vi "Sequence.BuildWaveform.vi"(10 "Steps":string[][](array[string]), 11 "Duration":string[](array[string])) -> (3 "Array":waveform(dbl)[](array[waveform]))   [LabVIEW 2013, in "Simple Sequence Tools - Shared.lvlib"]
uses:
  Simple Sequence Tools - Shared.lvlib
  <vilib>/Analysis/1siggen.llb/Ramp Pattern by Samples.vi
  <vilib>/Analysis/1siggen.llb/Ramp Pattern by Delta.vi
  <vilib>/Analysis/NI_AALBase.lvlib
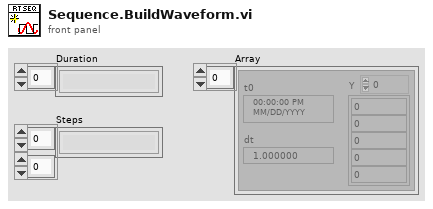
[diagram p1: front panel]
types:
  T1 = typedef "Simple Sequence Tools - Shared.lvlib/StepTypes.ctl" = enum8{"Step", "iStep", "Ramp", "Unchanged", "Unknown"}
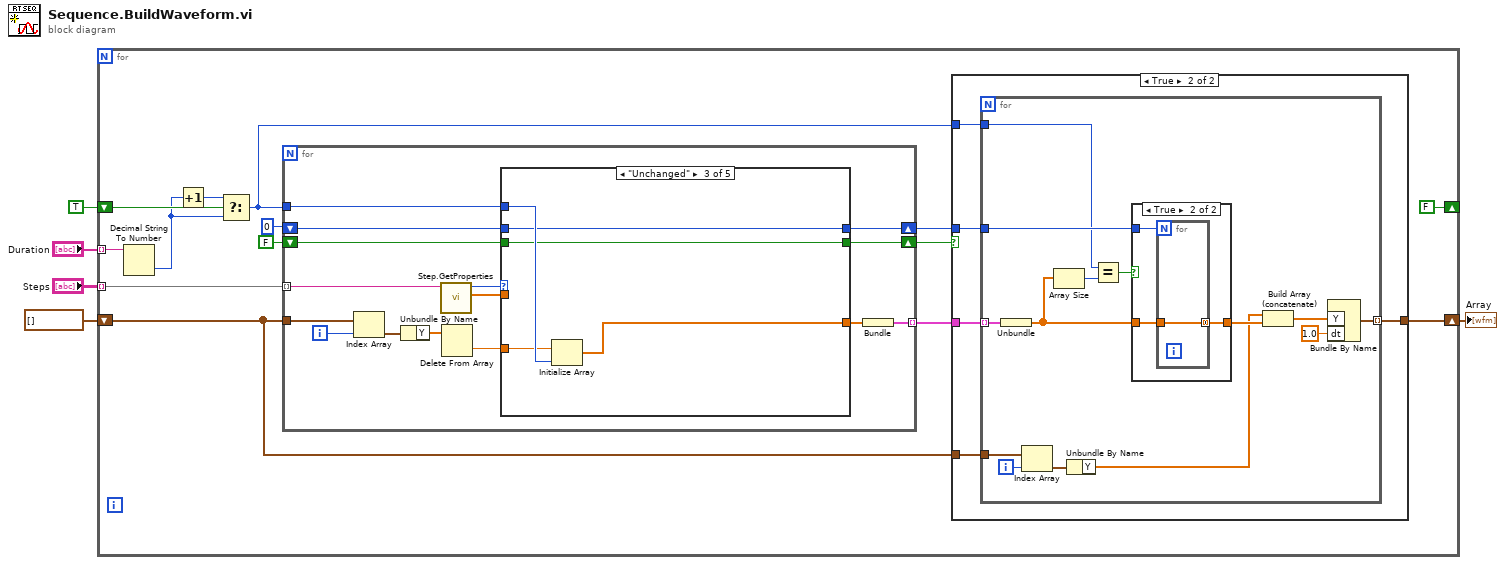
[diagram p0: block diagram]
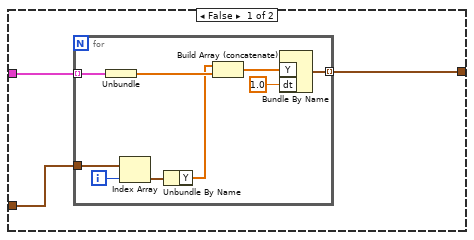
[diagram p2: hidden frame]
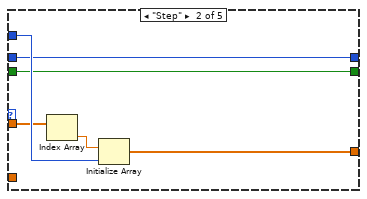
[diagram p5: hidden frame]
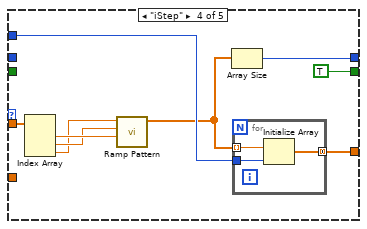
[diagram p6: hidden frame]
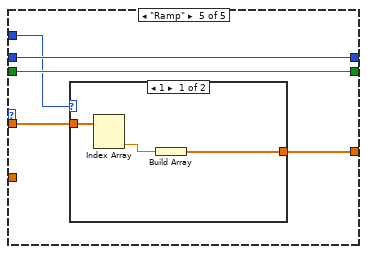
[diagram p7: hidden frame]
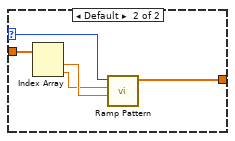
[diagram p8: hidden frame]
diagram:
  n1 = for {
    tunnel: "Steps" -> [w19] mode=indexing
    tunnel: "Duration" -> [w18] mode=indexing
    shift-right: [FALSE] -> _
    shift-left: TRUE -> [w11]
    shift-right: [w7] -> w1
    shift-left: waveform(dbl)[] [] -> [w6]
    n2 = Decimal String To Number(string=w18) -> (number=w10:i32)  [unwired: 2 in, 1 out]
    n3 = Increment(x=w10) -> (x+1=w9:i32)
    n4 = Select(t=w9, s=w11, f=w10) -> (s? t:f=w8:i32)
    n5 = for {
      tunnel: w19 -> [w70] mode=indexing
      tunnel: w8 -> [w68]
      shift-right: [w65] -> w15
      shift-left: FALSE -> [w66]
      shift-right: [w63] -> w14
      shift-left: 0 -> [w62]
      tunnel: [w61] -> w13 mode=indexing
      tunnel: w6 -> [w60]
      i -> [w58]
      n6 = Index Array(array=w60, index=w58) -> (element=w57:waveform(dbl))
      n7 = Unbundle By Name(w57) -> ("Y"=w56:dbl[])
      n8 = call "Step.GetProperties.vi"("String in"=w70) -> ("Parameters"=w67:dbl[], "Step"=w69:T1)  [unwired: 8 in, 1 out]
      n9 = Delete From Array(array=w56) -> (deleted portion=w59:dbl)  [unwired: 2 in, 1 out]
      n10 = case shown="\"Unchanged\"" w69 {
        tunnel: w68 -> [_ w78 w83 w91 w96]
        tunnel: w67 -> [_ w77 _ w92 w100]
        tunnel: [_ w75 w82 w86 w99] -> w64
        tunnel: w66 -> [w72 w74 w81 _ w98]
        tunnel: [w72 w74 w81 TRUE w98] -> w65
        tunnel: [w71 w73 w80 w84 w97] -> w63
        tunnel: w62 -> [w71 w73 w80 _ w97]
        tunnel: w59 -> [_ _ w79 _ _]
        frame Default {
        }
        frame "Step" {
          n11 = Index Array(array=w77) -> (element=w76:dbl)  [unwired: 1 in]
          n12 = Initialize Array(w76, w78) -> (w75:dbl[])
        }
        frame "Unchanged" {
          n13 = Initialize Array(w79, w83) -> (w82:dbl[])
        }
        frame "iStep" {
          n14 = Index Array(array=w92) -> (element #1=w90:dbl, element #2=w89:dbl, element #3=w88:dbl)  [unwired: 3 in]
          n15 = call-poly <vilib>:"Ramp Pattern.vi"("start"=w90, "end"=w89, "delta"=w88) -> ("Ramp Pattern"=w85:dbl[])  [unwired: 6 in, 2 out]
          n16 = Array Size(array=w85) -> (size(s)=w84:i32)
          n17 = for {
            tunnel: w91 -> [w95]
            tunnel: w85 -> [w94] mode=indexing
            tunnel: [w93] -> w86 mode=concatenating
            n18 = Initialize Array(w94, w95) -> (w93:dbl[])
          }
        }
        frame "Ramp" {
          n19 = case shown="1" w96 {
            selector: w96 -> [_ w104]
            tunnel: w100 -> [w103 w108]
            tunnel: [w101 w105] -> w99
            frame 1 {
              n20 = Index Array(array=w103) -> (element #2=w102:dbl)  [unwired: 2 in, 1 out]
              n21 = Build Array(w102) -> (w101:dbl[])
            }
            frame Default {
              n22 = Index Array(array=w108) -> (element #1=w107:dbl, element #2=w106:dbl)  [unwired: 2 in]
              n23 = call-poly <vilib>:"Ramp Pattern.vi"("start"=w107, "end"=w106, "samples"=w104) -> ("Ramp Pattern"=w105:dbl[])  [unwired: 7 in, 1 out]
            }
          }
        }
      }
      n24 = Bundle("Ramp Pattern"=w64) -> (w61:cluster{"Ramp Pattern":dbl[]})  [unwired: 1 in]
    }
    n25 = case shown="True" w15 {
      tunnel: w14 -> [_ w35]
      tunnel: w13 -> [w22 w36]
      tunnel: w8 -> [_ w34]
      tunnel: [w21 w33] -> w7
      tunnel: w6 -> [w20 w32]
      frame False {
        n26 = for {
          tunnel: w22 -> [w31] mode=indexing
          tunnel: [w29] -> w21 mode=indexing
          tunnel: w20 -> [w24]
          i -> [w25]
          n27 = Unbundle(w31) -> ("Ramp Pattern"=w28:dbl[])
          n28 = Index Array(array=w24, index=w25) -> (element=w23:waveform(dbl))
          n29 = Unbundle By Name(w23) -> ("Y"=w26:dbl[])
          n30 = Build Array (concatenate)(w26, w28) -> (w27:dbl[])
          n31 = Bundle By Name("Y"=w27, "dt"=1.0) -> (w29:waveform(dbl))  [unwired: 1 in]
        }
      }
      frame True {
        n32 = for {
          tunnel: w36 -> [w49] mode=indexing
          tunnel: w35 -> [w50]
          tunnel: w34 -> [w46]
          tunnel: [w43] -> w33 mode=indexing
          tunnel: w32 -> [w38]
          i -> [w39]
          n33 = Unbundle(w49) -> ("Ramp Pattern"=w48:dbl[])
          n34 = Index Array(array=w38, index=w39) -> (element=w37:waveform(dbl))
          n35 = Array Size(array=w48) -> (size(s)=w47:i32)
          n36 = Unbundle By Name(w37) -> ("Y"=w40:dbl[])
          n37 = Equal?(x=w46, y=w47) -> (x = y?=w45:bool)
          n38 = case shown="True" w45 {
            tunnel: w50 -> [_ w54]
            tunnel: w48 -> [w51 w53]
            tunnel: [w51 w52] -> w42
            frame False {
            }
            frame True {
              n39 = for {
                N: w54 -> [_]
                tunnel: w53 -> [w55]
                tunnel: [w55] -> w52 mode=concatenating
              }
            }
          }
          n40 = Build Array (concatenate)(w40, w42) -> (w41:dbl[])
          n41 = Bundle By Name("Y"=w41, "dt"=1.0) -> (w43:waveform(dbl))  [unwired: 1 in]
        }
      }
    }
  }
  "Array" <- w1
